vi "Begin.vi"(8 "error in":errorcluster) -> (0 "error out":errorcluster)   [LabVIEW 2015]
doc: "Called before other user functions, this VI is expected to open initial I/O refnums, load in file data, and do all program initialization. Notice that the <B>error out</B> terminal is simply used for data flow. Wiring it to other structures or subVIs ensures that this VI runs first."
uses:
  <vilib>/Rock Robotics/WPI/Joystick/WPI_JoystickDeviceEnum.ctl
  <vilib>/Rock Robotics/WPI/CAN/TalonSRX/WPI_CANTalonSRX_APIControlMode.ctl
  <vilib>/Rock Robotics/WPI/Solenoid/WPI_SolenoidChannel.ctl
  <vilib>/Rock Robotics/WPI/Solenoid/WPI_SolenoidValue.ctl
  <vilib>/Rock Robotics/SystemInterfaces/DIO/FPGA_DIOChannel.ctl
  <vilib>/Rock Robotics/WPI/CAN/TalonSRX/WPI_CANTalonSRX_StatusFrame.ctl
  <vilib>/Rock Robotics/SystemInterfaces/spilib/spi_bus.ctl
  <vilib>/Rock Robotics/SystemInterfaces/DIO/FPGA_DIOPWMChannel.ctl
  <vilib>/Rock Robotics/WPI/CAN/TalonSRX/WPI_CANTalonSRX_APIFeedbackSelect.ctl
  <vilib>/Rock Robotics/WPI/MotorControl/WPI_MotorControlOpenCANTalonSRX.vi
  <vilib>/Rock Robotics/WPI/Solenoid/WPI_SolenoidOpenSingle.vi
  <vilib>/Rock Robotics/WPI/Solenoid/WPI_SolenoidSetEnum.vi
  <vilib>/Rock Robotics/WPI/Switch/WPI_SwitchOpenLimit.vi
  <vilib>/Rock Robotics/WPI/Solenoid/WPI_SolenoidOpenDouble.vi
  RobotCode/MonitorGlobals.vi
  Utilities/AutoVars.vi
  navx-mxp/labview/navX Library v2/IO/Open/Z900_navX_Open_SPI.vi
  <vilib>/Rock Robotics/WPI/Utilities/WPI_GetSetVariantRefNum.vi
  navx-mxp/labview/navX Library v2/navX Library v2.lvlib
panel:
  in  "Climber PID Gains":T1={"proportional gain (Kc)"=3.0, "integral time (Ti, min)"=0.0, "derivative time (Td, min)"=7.0}
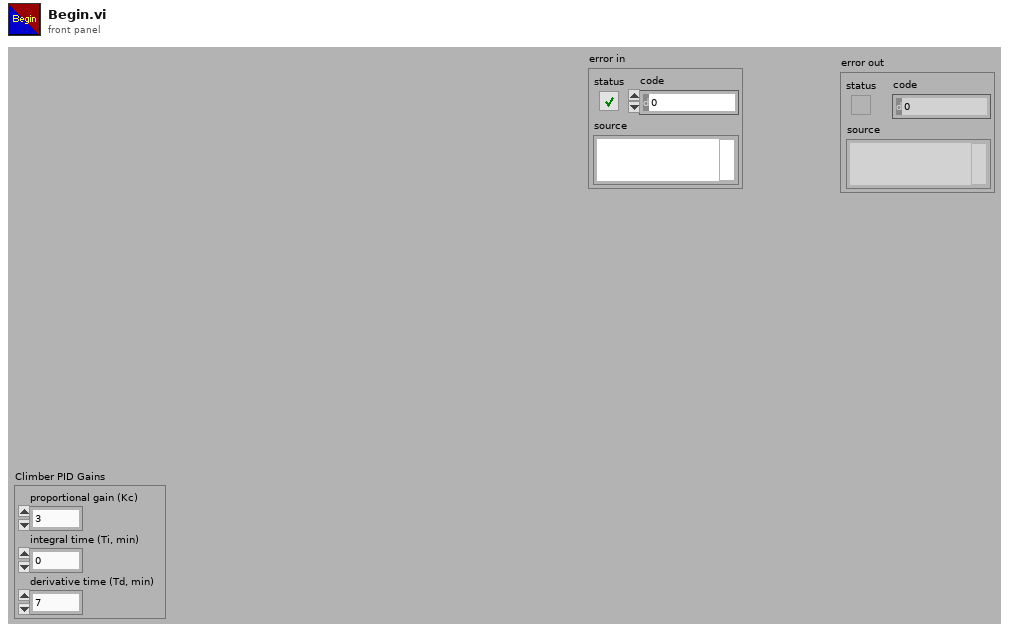
[diagram p1: front panel]
types:
  T1 = cluster{"proportional gain (Kc)":dbl, "integral time (Ti, min)":dbl, "derivative time (Td, min)":dbl}
  T2 = typedef "WPI_CANTalonSRX_APIFeedbackSelect.ctl" = enum16{"Digital Quadrature Encoder", "Analog Potentiometer", "Analog Encoder", "Count on Quad-A (Rising-Edge)", "Count on Quad-A (Falling-Edge)", "CTR Magnetic Enc (Absolute)", "CTR Magnetic Enc (Relative)", "Pulse Width"}
  T3 = typedef "WPI_CANTalonSRX_APIControlMode.ctl" = enum8{"Percent VBus", "Speed", "Position", "Slave", "Unchanged / Invalid", "Voltage Compensation", "Current", "Motion Profile"}
  T4 = typedef "WPI_CANTalonSRX_StatusFrame.ctl" = enum16{"General Status Frame", "Feedback Status Frame", "Quadrature Status Frame", "Analog Temp Vbat Status Frame", "Pulse Width Status Frame"}
  T5 = typedef "FPGA_DIOChannel.ctl" = enum8{"DIO 0", "DIO 1", "DIO 2", "DIO 3", "DIO 4", "DIO 5", "DIO 6", "DIO 7", "DIO 8", "DIO 9", "DIO MXP 0", "DIO MXP 1", "DIO MXP 2", "DIO MXP 3", "DIO MXP 4", "DIO MXP 5", "DIO MXP 6", "DIO MXP 7", "DIO MXP 8", "DIO MXP 9", "DIO MXP 10", "DIO MXP 11", "DIO MXP 12", "DIO MXP 13", "DIO MXP 14", "DIO MXP 15", "Invalid"}
  T6 = typedef "FPGA_DIOPWMChannel.ctl" = enum8{"PWM 0", "PWM 1", "PWM 2", "PWM 3", "PWM 4", "PWM 5", "PWM 6", "PWM 7", "PWM 8", "PWM 9", "PWM MXP 0", "PWM MXP 1", "PWM MXP 2", "PWM MXP 3", "PWM MXP 4", "PWM MXP 5", "PWM MXP 6", "PWM MXP 7", "PWM MXP 8", "PWM MXP 9", "Invalid"}
  T7 = typedef "spi_bus.ctl" = enum16{"SPI On-Board, CS0", "SPI On-Board, CS1", "SPI On-Board, CS2", "SPI On-Board, CS3", "SPI MXP", "Invalid"}
  T8 = typedef "WPI_SolenoidChannel.ctl" = enum8{"Solenoid 0", "Solenoid 1", "Solenoid 2", "Solenoid 3", "Solenoid 4", "Solenoid 5", "Solenoid 6", "Solenoid 7", "Invalid"}
  T9 = typedef "WPI_SolenoidValue.ctl" = enum16{"Off", "On", "Forward", "Reverse"}
  T10 = typedef "WPI_JoystickDeviceEnum.ctl" = enum16{"USB 0", "USB 1", "USB 2", "USB 3", "USB 4", "USB 5"}
  T11 = typedef "WPI_CompressorDevRef.ctl" = cluster{"DevStatus":errorcluster, "Pneumatics Control Module":u8}
  T12 = typedef "WPI_JoystickDevRef.ctl" = cluster{"Device":T10}
  T13 = typedef "WPI_DigitalOutputDevRef.ctl" = cluster{"DIO Channel":T5, "DevStatus":errorcluster}
  T14 = typedef "WPI_SwitchDevRef.ctl" = cluster{"DevStatus":errorcluster, "DIO Channel":T5, "CntIndex":T15, "Normally Closed":bool}
  T15 = typedef "FPGA_CounterCtrSystemIndex.ctl" = enum8{"Ctr 0", "Ctr 1", "Ctr 2", "Ctr 3", "Ctr 4", "Ctr 5", "Ctr 6", "Ctr 7", "Invalid"}
  T16 = typedef "WPI_SolenoidDevRef.ctl" = cluster{"DevStatus":errorcluster, "Pneumatics Control Module":u8, "Forward Solenoid Channel":T8, "Reverse Solenoid Channel":T8}
  T17 = typedef "WPI_ServoDeviceRef.ctl" = cluster{"DeviceStatus":errorcluster, "PWM Channel":T6, "DeadBand":T18}
  T18 = typedef "WPI_PWMDeadband.ctl" = cluster{"Name":string, "maxPositivePwm":i32, "minPositivePwm":i32, "centerPwm":i32, "maxNegativePwm":i32, "minNegativePwm":i32, "angularRange":u16}
  T19 = typedef "navX Library v2.lvlib/Z900_navX_DeviceTypeDef.ctl" = cluster{"Interface":cluster{"Protocol":T20, "Update Rate (4Hz-100Hz)":u8, "navX Open TypeDef":variant}, "Notify Packet":refnum<notifier>, "Loop VI Refnum":refnum<vi>, "Ready to Close Occurrence Refnum":refnum<k4>}
  T20 = typedef "navX Library v2.lvlib/Z900_navX_ProtocolTypeDef.ctl" = enum16{"SERIAL", "I2C", "SPI"}
  T21 = typedef "WPI_MotorControlDeviceRef.ctl" = cluster{"DeviceStatus":errorcluster, "Type":T22, "PWM":cluster{"PWM Channel":T6, "DeadBand":T18}, "CAN":cluster{"Device Number":u8, "Control Mode":T23, "Semaphore":T24, "Max Vout":dbl, "TalonSRX Control Mode":T3}, "Invert":bool}
  T22 = typedef "WPI_MotorControlType.ctl" = enum16{"PWM", "CAN", "CANTalonSRX"}
  T23 = typedef "WPI_CANJaguar_ControlMode.ctl" = enum8{"Percent VBus", "Current", "Speed", "Position", "Voltage"}
  T24 = typedef "Semaphore RefNum" = refnum<k1>
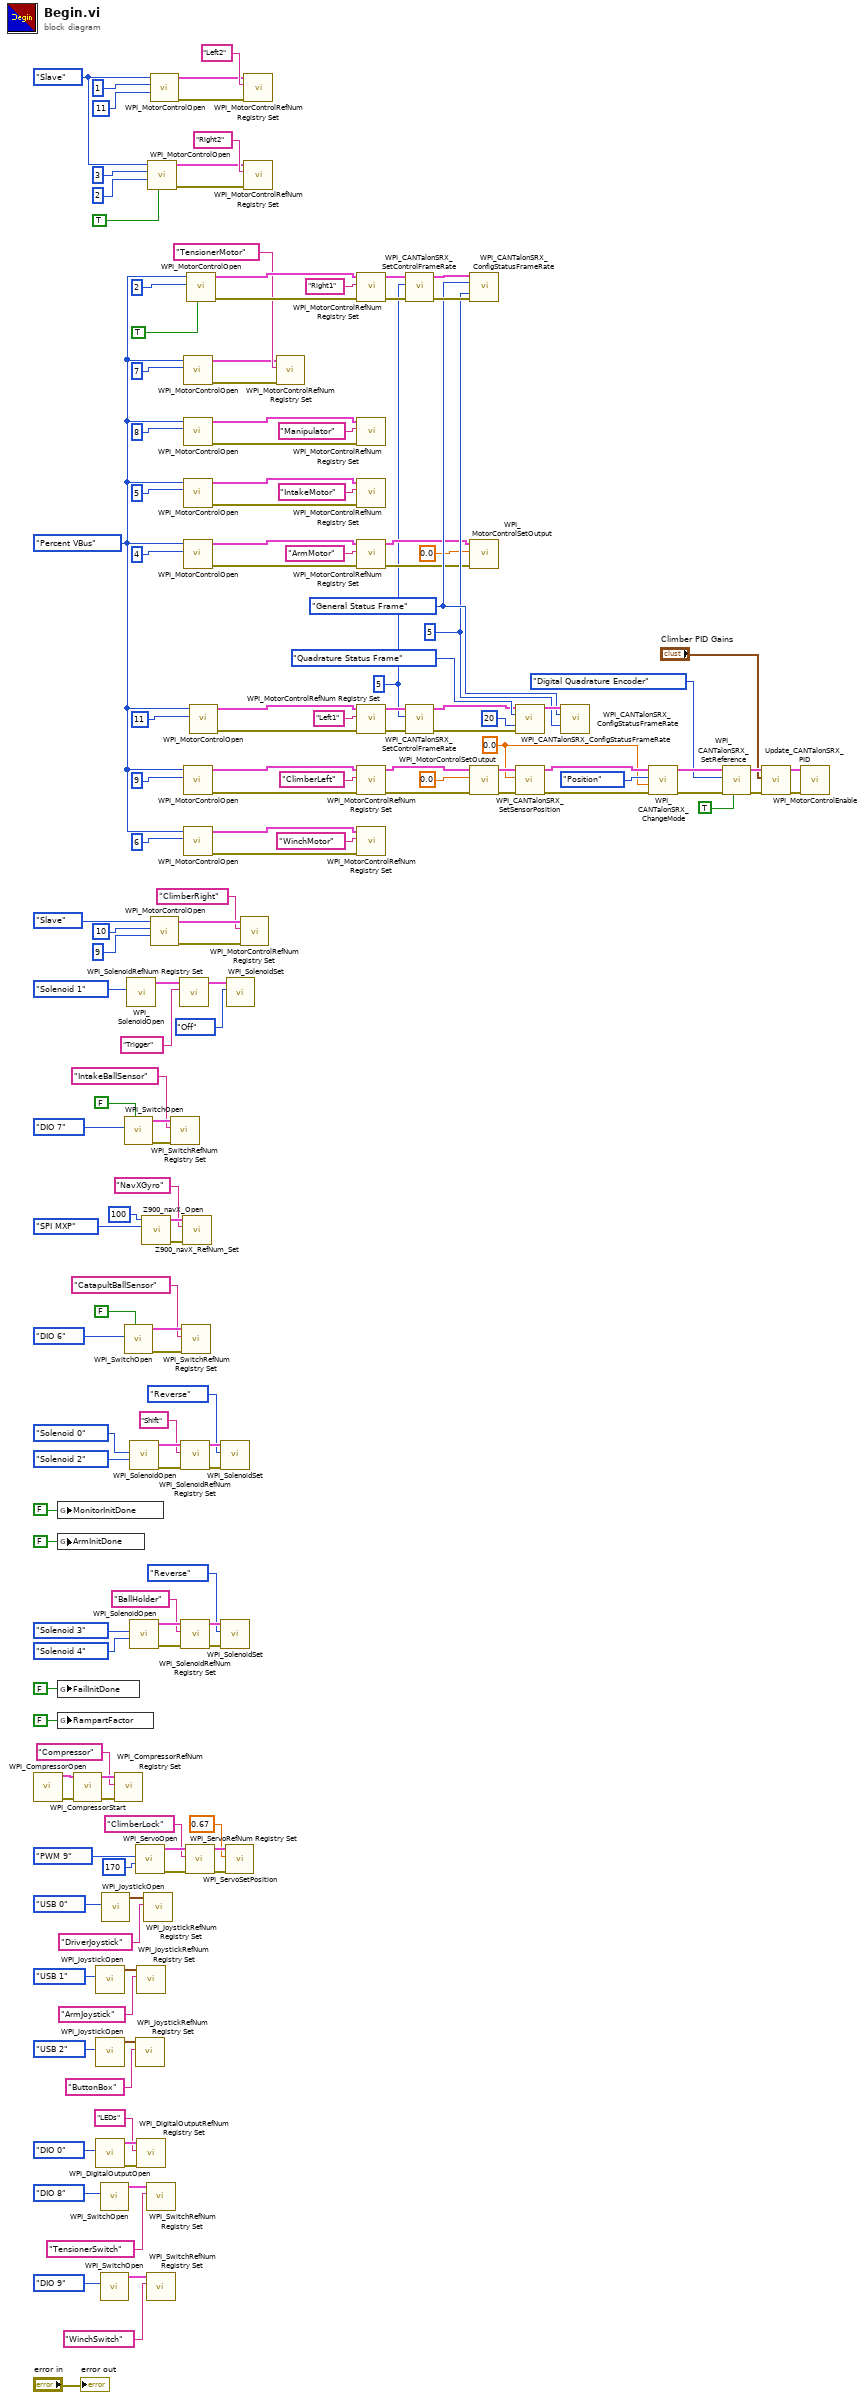
[diagram p0: block diagram]
diagram:
  w1 = 0.0 ("Encoder Initial Position")
  w23 = u32 5 ("Frame Rate Ms")
  w24 = WPI_CANTalonSRX_StatusFrame."General Status Frame" ("Talon SRX Status Frame")
  w19 = u8 5 ("Control Frame Rate (ms)")
  w81 = WPI_CANTalonSRX_APIControlMode."Slave" ("Control Mode")
  w83 = WPI_CANTalonSRX_APIControlMode."Percent VBus" ("Control Mode")
  n1 = call <vilib>:"WPI_CompressorOpen.vi"() -> ("CompressorDevRef"=w147:T11, "error out"=w146:errorcluster)  [unwired: 14 in]
  n2 = global write "MonitorGlobals.vi" "MonitorInitDone"(FALSE ("MonitorInitDone")) -> ()
  n3 = global write "AutoVars.vi" "ArmInitDone"(FALSE ("ArmInitDone")) -> ()
  n4 = global write "AutoVars.vi" "FailInitDone"(FALSE ("InitDone")) -> ()
  n5 = global write "AutoVars.vi" "RampartFactor"(FALSE ("InitDone")) -> ()
  n6 = call <vilib>:"WPI_CompressorStart.vi"("error in (no error)"=w146, "CompressorDevRef"=w147) -> ("error out"=w149:errorcluster, "CompressorDevRef"=w148:T11)  [unwired: 8 in]
  n7 = call <vilib>:"WPI_JoystickOpen.vi"("JoystickDevice"=WPI_JoystickDeviceEnum."USB 1") -> ("JoystickDevRef"=w138:T12)  [unwired: 10 in]
  n8 = call <vilib>:"WPI_JoystickOpen.vi"("JoystickDevice"=WPI_JoystickDeviceEnum."USB 2") -> ("JoystickDevRef"=w125:T12)  [unwired: 10 in]
  n9 = call <vilib>:"WPI_DigitalOutputOpen.vi"("DIO Channel"=FPGA_DIOChannel."DIO 0") -> ("error out"=w121:errorcluster, "DigitalOutputDevRef"=w122:T13)  [unwired: 9 in]
  n10 = call-poly <vilib>:"WPI_SwitchOpen.vi"("DIO Channel"=FPGA_DIOChannel."DIO 8") -> ("SwitchDevRef"=w131:T14)  [unwired: 9 in, 1 out]
  n11 = call-poly <vilib>:"WPI_SwitchOpen.vi"("DIO Channel"=FPGA_DIOChannel."DIO 9") -> ("SwitchDevRef"=w128:T14)  [unwired: 9 in, 1 out]
  n12 = call <vilib>:"WPI_JoystickOpen.vi"("JoystickDevice"=WPI_JoystickDeviceEnum."USB 0") -> ("JoystickDevRef"=w160:T12)  [unwired: 10 in]
  n13 = call <vilib>:"WPI_CompressorRefNum Registry Set.vi"("error in (no error)"=w149, "refnum name"="Compressor", "CompressorDevRef"=w148) -> ()  [unwired: 7 in, 2 out]
  n14 = call-poly <vilib>:"WPI_SwitchOpen.vi"("Normally Closed"=FALSE, "DIO Channel"=FPGA_DIOChannel."DIO 7") -> ("error out"=w93:errorcluster, "SwitchDevRef"=w94:T14)  [unwired: 8 in]
  n15 = call-poly <vilib>:"WPI_SwitchOpen.vi"("Normally Closed"=FALSE, "DIO Channel"=FPGA_DIOChannel."DIO 6") -> ("error out"=w88:errorcluster, "SwitchDevRef"=w89:T14)  [unwired: 8 in]
  n16 = call-poly <vilib>:"WPI_SolenoidOpen.vi"("Solenoid Channel"=WPI_SolenoidChannel."Solenoid 1") -> ("SolenoidDevRef"=w136:T16)  [unwired: 9 in, 1 out]
  n17 = call-poly <vilib>:"WPI_SolenoidOpen.vi"("Reverse Solenoid Channel"=WPI_SolenoidChannel."Solenoid 2", "Forward Solenoid Channel"=WPI_SolenoidChannel."Solenoid 0" ("Solenoid Channel")) -> ("error out"=w155:errorcluster, "SolenoidDevRef"=w154:T16)  [unwired: 8 in]
  n18 = call-poly <vilib>:"WPI_SolenoidOpen.vi"("Reverse Solenoid Channel"=WPI_SolenoidChannel."Solenoid 4", "Forward Solenoid Channel"=WPI_SolenoidChannel."Solenoid 3" ("Solenoid Channel")) -> ("error out"=w115:errorcluster, "SolenoidDevRef"=w116:T16)  [unwired: 8 in]
  n19 = call <vilib>:"WPI_ServoOpen.vi"("Angular Range"=u16 170, "PWM Channel"=FPGA_DIOPWMChannel."PWM 9") -> ("error out"=w99:errorcluster, "ServoDeviceRef"=w98:T17)  [unwired: 8 in]
  n20 = call <vilib>:"WPI_JoystickRefNum Registry Set.vi"("refnum name"="ButtonBox", "JoystickDevRef"=w125) -> ()  [unwired: 8 in, 2 out]
  n21 = call <vilib>:"WPI_JoystickRefNum Registry Set.vi"("refnum name"="ArmJoystick", "JoystickDevRef"=w138) -> ()  [unwired: 8 in, 2 out]
  n22 = call <vilib>:"WPI_DigitalOutputRefNum Registry Set.vi"("error in (no error)"=w121, "refnum name"="LEDs", "DigitalOutputDevRef"=w122) -> ()  [unwired: 7 in, 2 out]
  n23 = call-poly "Z900_navX_Open.vi"("SPI Bus"=spi_bus."SPI MXP", "Update Rate (4Hz-60Hz)"=u8 100) -> ("error out"=w105:errorcluster, "navX Device"=w106:T19)  [unwired: 8 in]
  n24 = call <vilib>:"WPI_JoystickRefNum Registry Set.vi"("refnum name"="DriverJoystick", "JoystickDevRef"=w160) -> ()  [unwired: 8 in, 2 out]
  n25 = call <vilib>:"WPI_SwitchRefNum Registry Set.vi"("refnum name"="TensionerSwitch", "SwitchDevRef"=w131) -> ()  [unwired: 8 in, 2 out]
  n26 = call <vilib>:"WPI_SwitchRefNum Registry Set.vi"("refnum name"="WinchSwitch", "SwitchDevRef"=w128) -> ()  [unwired: 8 in, 2 out]
  n27 = call-poly <vilib>:"WPI_MotorControlOpen.vi"("Invert"=TRUE, "Master Device Number"=u8 2, "Device Number"=u8 3, "Control Mode"=w81) -> ("error out"=w74:errorcluster, "MotorControlDeviceRef"=w73:T21)  [unwired: 6 in]
  n28 = call-poly <vilib>:"WPI_MotorControlOpen.vi"("Master Device Number"=u8 11, "Device Number"=u8 1, "Control Mode"=w81) -> ("error out"=w79:errorcluster, "MotorControlDeviceRef"=w78:T21)  [unwired: 7 in]
  n29 = call-poly <vilib>:"WPI_MotorControlOpen.vi"("Master Device Number"=u8 9, "Device Number"=u8 10, "Control Mode"=WPI_CANTalonSRX_APIControlMode."Slave") -> ("error out"=w32:errorcluster, "MotorControlDeviceRef"=w33:T21)  [unwired: 7 in]
  n30 = call <vilib>:"WPI_SwitchRefNum Registry Set.vi"("error in (no error)"=w93, "refnum name"="IntakeBallSensor", "SwitchDevRef"=w94) -> ()  [unwired: 7 in, 2 out]
  n31 = call <vilib>:"WPI_SolenoidRefNum Registry Set.vi"("refnum name"="Trigger", "SolenoidDevRef"=w136) -> ("SolenoidDevRef"=w134:T16)  [unwired: 8 in, 1 out]
  n32 = call <vilib>:"WPI_SolenoidRefNum Registry Set.vi"("error in (no error)"=w155, "refnum name"="Shift", "SolenoidDevRef"=w154) -> ("error out"=w151:errorcluster, "SolenoidDevRef"=w152:T16)  [unwired: 7 in]
  n33 = call <vilib>:"WPI_SolenoidRefNum Registry Set.vi"("error in (no error)"=w115, "refnum name"="BallHolder", "SolenoidDevRef"=w116) -> ("error out"=w117:errorcluster, "SolenoidDevRef"=w118:T16)  [unwired: 7 in]
  n34 = call <vilib>:"WPI_SwitchRefNum Registry Set.vi"("error in (no error)"=w88, "refnum name"="CatapultBallSensor", "SwitchDevRef"=w89) -> ()  [unwired: 7 in, 2 out]
  n35 = call "Z900_navX_RefNum_Set.vi"("error in (no error)"=w105, "refnum name"="NavXGyro", "navX Device"=w106) -> ()  [unwired: 7 in, 2 out]
  n36 = call-poly <vilib>:"WPI_MotorControlOpen.vi"("Device Number"=u8 7, "Control Mode"=w83) -> ("error out"=w44:errorcluster, "MotorControlDeviceRef"=w45:T21)  [unwired: 8 in]
  n37 = call-poly <vilib>:"WPI_MotorControlOpen.vi"("Device Number"=u8 8, "Control Mode"=w83) -> ("error out"=w52:errorcluster, "MotorControlDeviceRef"=w53:T21)  [unwired: 8 in]
  n38 = call-poly <vilib>:"WPI_MotorControlOpen.vi"("Device Number"=u8 5, "Control Mode"=w83) -> ("error out"=w58:errorcluster, "MotorControlDeviceRef"=w57:T21)  [unwired: 8 in]
  n39 = call-poly <vilib>:"WPI_MotorControlOpen.vi"("Device Number"=u8 4, "Control Mode"=w83) -> ("error out"=w141:errorcluster, "MotorControlDeviceRef"=w144:T21)  [unwired: 8 in]
  n40 = call-poly <vilib>:"WPI_MotorControlOpen.vi"("Device Number"=u8 9, "Control Mode"=w83) -> ("error out"=w49:errorcluster, "MotorControlDeviceRef"=w50:T21)  [unwired: 8 in]
  n41 = call-poly <vilib>:"WPI_MotorControlOpen.vi"("Device Number"=u8 6, "Control Mode"=w83) -> ("error out"=w67:errorcluster, "MotorControlDeviceRef"=w68:T21)  [unwired: 8 in]
  n42 = call <vilib>:"WPI_ServoRefNum Registry Set.vi"("error in (no error)"=w99, "refnum name"="ClimberLock", "ServoDeviceRef"=w98) -> ("error out"=w95:errorcluster, "ServoDeviceRef"=w96:T17)  [unwired: 7 in]
  n43 = call-poly <vilib>:"WPI_MotorControlOpen.vi"("Invert"=TRUE, "Device Number"=u8 2, "Control Mode"=w83) -> ("error out"=w64:errorcluster, "MotorControlDeviceRef"=w59:T21)  [unwired: 7 in]
  n44 = call-poly <vilib>:"WPI_MotorControlOpen.vi"("Device Number"=u8 11, "Control Mode"=w83) -> ("error out"=w40:errorcluster, "MotorControlDeviceRef"=w41:T21)  [unwired: 8 in]
  n45 = call-poly <vilib>:"WPI_SolenoidSet.vi"("error in (no error)"=w151, "Value"=WPI_SolenoidValue."Reverse", "SolenoidDevRef"=w152) -> ()  [unwired: 7 in, 2 out]
  n46 = call-poly <vilib>:"WPI_SolenoidSet.vi"("error in (no error)"=w117, "Value"=WPI_SolenoidValue."Reverse", "SolenoidDevRef"=w118) -> ()  [unwired: 7 in, 2 out]
  n47 = call <vilib>:"WPI_ServoSetPosition.vi"("error in (no error)"=w95, "Position"=0.67, "ServoDeviceRef"=w96) -> ()  [unwired: 7 in, 2 out]
  n48 = call-poly <vilib>:"WPI_SolenoidSet.vi"("Value"=WPI_SolenoidValue."Off", "SolenoidDevRef"=w134) -> ()  [unwired: 8 in, 2 out]
  n49 = call <vilib>:"WPI_MotorControlRefNum Registry Set.vi"("error in (no error)"=w32, "refnum name"="ClimberRight", "MotorControlDevRef"=w33) -> ()  [unwired: 7 in, 2 out]
  n50 = call <vilib>:"WPI_MotorControlRefNum Registry Set.vi"("error in (no error)"=w79, "refnum name"="Left2", "MotorControlDevRef"=w78) -> ()  [unwired: 7 in, 2 out]
  n51 = call <vilib>:"WPI_MotorControlRefNum Registry Set.vi"("error in (no error)"=w74, "refnum name"="Right2", "MotorControlDevRef"=w73) -> ()  [unwired: 7 in, 2 out]
  n52 = call <vilib>:"WPI_MotorControlRefNum Registry Set.vi"("error in (no error)"=w44, "refnum name"="TensionerMotor", "MotorControlDevRef"=w45) -> ()  [unwired: 7 in, 2 out]
  n53 = call <vilib>:"WPI_MotorControlRefNum Registry Set.vi"("error in (no error)"=w64, "refnum name"="Right1", "MotorControlDevRef"=w59) -> ("error out"=w60:errorcluster, "MotorControlDevRef"=w61:T21)  [unwired: 7 in]
  n54 = call <vilib>:"WPI_MotorControlRefNum Registry Set.vi"("error in (no error)"=w52, "refnum name"="Manipulator", "MotorControlDevRef"=w53) -> ()  [unwired: 7 in, 2 out]
  n55 = call <vilib>:"WPI_MotorControlRefNum Registry Set.vi"("error in (no error)"=w58, "refnum name"="IntakeMotor", "MotorControlDevRef"=w57) -> ()  [unwired: 7 in, 2 out]
  n56 = call <vilib>:"WPI_MotorControlRefNum Registry Set.vi"("error in (no error)"=w141, "refnum name"="ArmMotor", "MotorControlDevRef"=w144) -> ("error out"=w22:errorcluster, "MotorControlDevRef"=w21:T21)  [unwired: 7 in]
  n57 = call <vilib>:"WPI_MotorControlRefNum Registry Set.vi"("error in (no error)"=w40, "refnum name"="Left1", "MotorControlDevRef"=w41) -> ("error out"=w37:errorcluster, "MotorControlDevRef"=w38:T21)  [unwired: 7 in]
  n58 = call <vilib>:"WPI_MotorControlRefNum Registry Set.vi"("error in (no error)"=w49, "refnum name"="ClimberLeft", "MotorControlDevRef"=w50) -> ("error out"=w17:errorcluster, "MotorControlDevRef"=w18:T21)  [unwired: 7 in]
  n59 = call <vilib>:"WPI_MotorControlRefNum Registry Set.vi"("error in (no error)"=w67, "refnum name"="WinchMotor", "MotorControlDevRef"=w68) -> ()  [unwired: 7 in, 2 out]
  n60 = call <vilib>:"WPI_CANTalonSRX_SetControlFrameRate.vi"("error in (no error)"=w60, "Control Frame Rate (ms)"=w19, "CAN Talon SRX Ref"=w61) -> ("error out"=w25:errorcluster, "CAN Talon SRX Ref"=w26:T21)  [unwired: 7 in]
  n61 = call <vilib>:"WPI_CANTalonSRX_SetControlFrameRate.vi"("error in (no error)"=w37, "Control Frame Rate (ms)"=w19, "CAN Talon SRX Ref"=w38) -> ("error out"=w35:errorcluster, "CAN Talon SRX Ref"=w36:T21)  [unwired: 7 in]
  n62 = call <vilib>:"WPI_CANTalonSRX_ConfigStatusFrameRate.vi"("CAN Talon SRX Ref"=w26, "Talon SRX Status Frame"=w24, "Frame Rate Ms"=w23, "error in (no error)"=w25) -> ()  [unwired: 11 in, 1 out]
  n63 = call <vilib>:"WPI_MotorControlSetOutput.vi"("error in (no error)"=w22, "Output"=0.0, "MotorControlDevRef"=w21) -> ()  [unwired: 6 in, 3 out]
  n64 = call <vilib>:"WPI_MotorControlSetOutput.vi"("error in (no error)"=w17, "Output"=0.0, "MotorControlDevRef"=w18) -> ("error out"=w2:errorcluster, "MotorControlDevRef"=w3:T21)  [unwired: 6 in, 1 out]
  n65 = call <vilib>:"WPI_CANTalonSRX_ConfigStatusFrameRate.vi"("CAN Talon SRX Ref"=w36, "Talon SRX Status Frame"=WPI_CANTalonSRX_StatusFrame."Quadrature Status Frame", "Frame Rate Ms"=u32 20, "error in (no error)"=w35) -> ("CAN Talon SRX Ref"=w27:T21)  [unwired: 11 in]
  n66 = call <vilib>:"WPI_CANTalonSRX_SetSensorPosition.vi"("error in (no error)"=w2, "New Sensor Position"=w1, "CAN Talon SRX Ref"=w3) -> ("error out"=w4:errorcluster, "CAN Talon SRX Ref"=w5:T21)  [unwired: 7 in]
  n67 = call <vilib>:"WPI_CANTalonSRX_ConfigStatusFrameRate.vi"("CAN Talon SRX Ref"=w27, "Talon SRX Status Frame"=w24, "Frame Rate Ms"=w23) -> ()  [unwired: 12 in, 1 out]
  n68 = call <vilib>:"WPI_CANTalonSRX_ChangeMode.vi"("error in (no error)"=w4, "Output"=w1, "Control Mode"=WPI_CANTalonSRX_APIControlMode."Position", "CAN Talon SRX Ref"=w5) -> ("error out"=w14:errorcluster, "CAN Talon SRX Ref"=w15:T21)  [unwired: 6 in]
  n69 = call <vilib>:"WPI_CANTalonSRX_SetReference.vi"("Reverse Closed-Loop Output"=TRUE, "error in (no error)"=w14, "Feedback Reference"=WPI_CANTalonSRX_APIFeedbackSelect."Digital Quadrature Encoder", "CAN Talon SRX Ref"=w15) -> ("error out"=w13:errorcluster, "CAN Talon SRX Ref"=w12:T21)  [unwired: 6 in]
  n70 = call "Update_CANTalonSRX_PID.vi"("error in (no error)"=w13, "PID Gains"="Climber PID Gains", "CAN Talon SRX Ref"=w12) -> ("error out"=w11:errorcluster, "CAN Talon SRX Ref Out"=w10:T21)  [unwired: 7 in]
  n71 = call <vilib>:"WPI_MotorControlEnable.vi"("error in (no error)"=w11, "CAN MotorDevRef"=w10) -> ()  [unwired: 8 in, 2 out]
  "error out" <- "error in"
